vi "UltraRead.vi"(4 "Reset":bool, 6 "UltrasonicParameters":T1={"MedianFilterSamples"=10, "LowPassFilterPercent"=0.0, "RailOffset (in)"=0.0, "MaxRange (in)"=0.0}, 7 "SonarMB1010DigitalDevRef":T2={"CounterDevRef"={"DevStatus"={"status"=FALSE, "code"=0, "source"=""}, "CntIndex"=enum."Invalid"}, "Scaling factor (s/in)"=0.0}) -> (1 "Unfiltered_UltrasonicRange (in)":dbl, 2 "MedianOnly_UltrasonicRange (in)":dbl, 3 "UltrasonicRange (in)":dbl)   [LabVIEW 2017, in "ArgosLib.lvlib"]
uses:
  ArgosLib.lvlib
  <vilib>/Rock Robotics/WPI/Ultrasonic/WPI_SonarMB1010DigitalDeviceRef.ctl
  <vilib>/Rock Robotics/WPI/Counter/WPI_CounterDevRef.ctl
  <vilib>/Rock Robotics/SystemInterfaces/Counter/FPGA_CounterCtrSystemIndex.ctl
  Ultrasonic/TypeDefs/UltrasonicParameters_Type.ctl
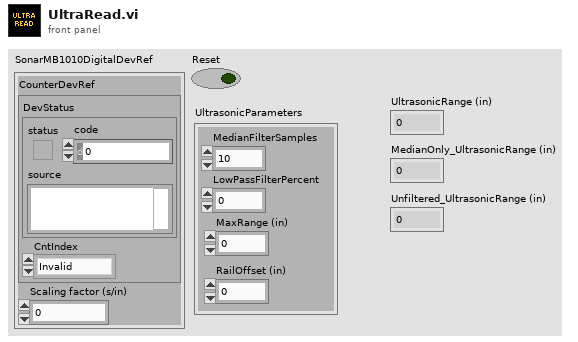
[diagram p1: front panel]
types:
  T1 = typedef "ArgosLib.lvlib/UltrasonicParameters_Type.ctl" = cluster{"MedianFilterSamples":u16, "LowPassFilterPercent":dbl, "RailOffset (in)":dbl, "MaxRange (in)":dbl}
  T2 = typedef "WPI_SonarMB1010DigitalDeviceRef.ctl" = cluster{"CounterDevRef":T3, "Scaling factor (s/in)":dbl}
  T3 = typedef "WPI_CounterDevRef.ctl" = cluster{"DevStatus":errorcluster, "CntIndex":T4}
  T4 = typedef "FPGA_CounterCtrSystemIndex.ctl" = enum8{"Ctr 0", "Ctr 1", "Ctr 2", "Ctr 3", "Ctr 4", "Ctr 5", "Ctr 6", "Ctr 7", "Invalid"}
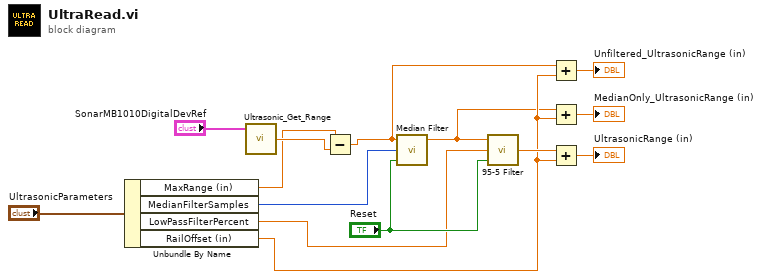
[diagram p0: block diagram]
diagram:
  n1 = Unbundle By Name("UltrasonicParameters") -> ("MaxRange (in)"=w1:dbl, "MedianFilterSamples"=w9:u16, "LowPassFilterPercent"=w8:dbl, "RailOffset (in)"=w4:dbl)
  n2 = call "Ultrasonic_Get_Range.vi"("SonarMB1010DigitalDevRef"="SonarMB1010DigitalDevRef") -> ("Range"=w2:dbl)  [unwired: 2 in, 2 out]
  n3 = Subtract(x=w1, y=w2) -> (x-y=w7:dbl)
  n4 = call "Median Filter.vi"("Reset"="Reset", "WindowSize"=w9, "Input"=w7) -> ("Output"=w3:dbl)  [unwired: 2 in]
  n5 = call "95-5 Filter.vi"("Reset"="Reset", "Percent"=w8, "In"=w3) -> ("Out"=w12:dbl)
  n6 = Add(x=w7, y=w4) -> (x+y=→"Unfiltered_UltrasonicRange (in)":dbl)
  n7 = Add(x=w3, y=w4) -> (x+y=→"MedianOnly_UltrasonicRange (in)":dbl)
  n8 = Add(x=w12, y=w4) -> (x+y=→"UltrasonicRange (in)":dbl)
